vi "AlliGator Update Settings Python Options & Valid Flag.vi"(8 "error in (no error)":errorcluster, 11 "Ctl Refnums":refnum<vi>[](array[refnum])) -> (0 "error out":errorcluster)   [LabVIEW 2021, in "AlliGator Settings.lvlib"]
doc: "Updates Python Plugins options and Valid Session flag in the Settings window."
uses:
  AlliGator Settings.lvlib
  AlliGator Python Settings.ctl
  AlliGator Variables List.ctl
  Variant/Variant to Data/Variant to Boolean.vi
  AlliGator Globals, Variables & Constants.lvlib
  Variant/Variant to Data/Variant to Data.lvlib
panel:
  out "Valid Python Session":bool
  in  "Python Settings":T1
  # "see the AlliGator License on the block diagram (Ctrl+E or Window:Show Block Diagram)"
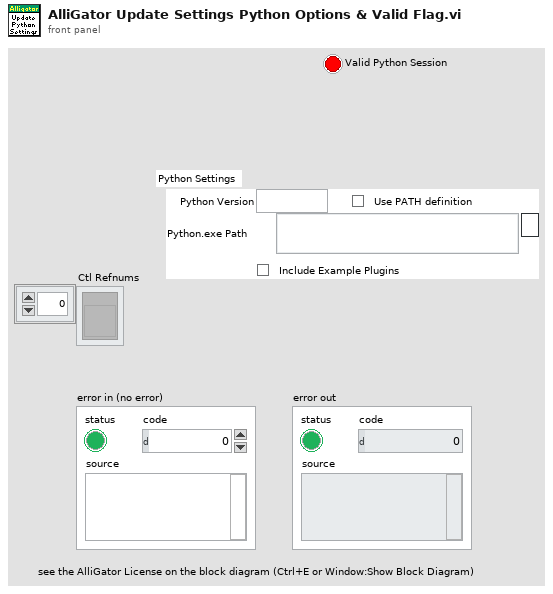
[diagram p1: front panel]
types:
  T1 = typedef "AlliGator Settings.lvlib/AlliGator Python Settings.ctl" = cluster{"Python Version":string, "Use PATH definition":bool, "Python.exe Path":path, "Include Example Plugins":bool}
  T2 = typedef "AlliGator Globals, Variables & Constants.lvlib/AlliGator Variables List.ctl" = enum16{"---- GUI ----", "Initialization Status", "State Indicators Refnum", "Original AlliGator Menu Items", "Current Action Loop State", "Script in progress", "Playback", "Loop Playback", "Search ROI Used", "Search ROI", "Decay Graph Max Legend Size", "Intensity Graph Max Legend Size", "Decay Statistics Graph Max Legend Size", "Phasor Graph Max Legend Size", "Phasor Ratio Graph Max Legend Size", "Lifetime Graph Max Legend Size", "---- Files ----", "Export Dataset Frames as Individual Files", "Show Batch Export Help Balloons", "Frames in Dataset", "ptu File Frame Start Indices", "Current Frame in Dataset", "Current Frame Timestamp", "------ Python Plugins ------", "Python Plugins Information", "Python Session", "Valid Python Session?", "---- Source Image ----", "Dataset Loaded", "Dataset Metadata", "Dataset Channel", "Dataset Data Description", "Background Dataset Metadata", "Background Dataset Channel", "Background Dataset Data Description", "Background File Subtraction", "Background File Path", "Background File Pile-up Correction", "Background File Pixel Well Capacity", "Background File Scaling Factor", "Source Image ROIs", "Current Source Image ROI", "Source Image ROI Event Refnum", "X_Source Image Display Range", "X_Source Image Palette Information", "Source Image Palette List", "Source Image Scale", "Current Dataset Load Settings", "Source Image:ROI Overlay Color", "---- Image Profile Window ----", "Image Profile:Overlay ROI in Source Image", "Image Profile Window Event Refnum", "Image Profile:IntensityType", "Image Profile:Intensity Average Type", "Image Profile:Intensity-weighted SDV", "Image Profile:Box Profile Type", "Image Profile Window Open", "Image Profile:Plotted Fit Parameter", "X_Type of Displayed Image", "X_Time Gate Slider", "Dataset Path", "Source Image Overlay to Erase", "Is Displayed Image Accumulated", "White Light Image Modified", "Mask Image Modified", "Macrotime Gate Separation", "------ Phasor Graph -------", "Phasor Graph:Show Line", "---- Phasor Plot ---", "Phasor Plot Parameters Changed", "FLI Dataset Modified since last Phasor Plot Calculation", "Phasor Harmonics Data", "Selected Phasor Harmonics", "Phasor Harmonic Manager Event Refnum", "Phasor Plot ROIs", "Current Phasor Plot ROI", "Phasor Plot ROI Event Refnum", "Phasor Plot Image Reference Points", "Phasor Plot Computed", "Phasor Plot Palette Information", "Phasor Plot Palette List", "Phasor Ratio Palette Information", "Phasor Ratio Palette List", "Phasor Image Scale", "Phasor Plot Image Overlay to Erase", "Phasor Plot Image Elements to Update", "Current Phasor Plot Calculation Parameters", "Current Phasor Calibration Options", "Reset Cumulated Phasor Plot", "Phasor Ratio Reference 1", "Phasor Ratio Lifetime Reference 1", "Phasor Ratio Reference 1 Frequency", "Phasor Ratio Reference 2", "Phasor Ratio Lifetime Reference 2", "Phasor Ratio Reference 2 Frequency", "---- Decay Analysis ----", "Number of Selected Decays to Fit", "LS Fit Results", "LAR Fit Results", "BS Fit Results", "Last Decay Max - Min", "Best Fit Parameters", "Best Fit Parameter Names", "Actual Size X", "Actual Size Y", "Binning X", "Binning Y", "Actual # Gates", "Dataset Number", "Gates to...", "Gates Skipped", "Gates to keep", "Gate Step", "Gate Separation", "Reversed Gates", "Pile-up Correction", "Pixel Well Capacity", "Background Subtracted", "Background Subtraction Method", "Background Definition Range", "Background File (deprecated)", "Number of Dataset Accumulated", "Array of Accumulated Dataset Paths", "Do Averaged Datasets", "Destination File Path", "Process Plot Target", "Use 1/D as Phasor Frequency", "---- Decay Fit Parameter Map -----", "Decay Fit Parameter Map Palette Information", "Decay Fit Parameter Map Palette List", "Local Decay Graph Window Event Refnum", "------- Local Decay Window ---------", "Use normalized IRF for convolution", "----- Miscellaneous ----", "Skippable Dialog Windows Status"}
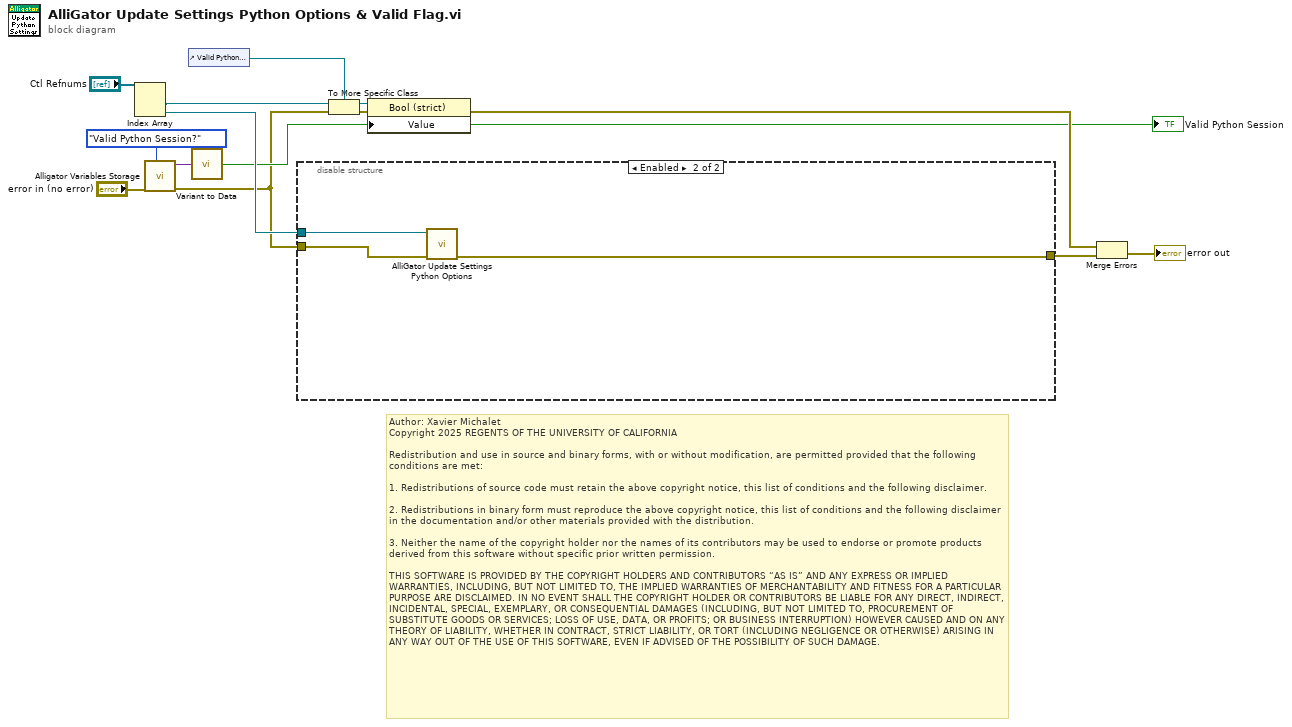
[diagram p0: block diagram]
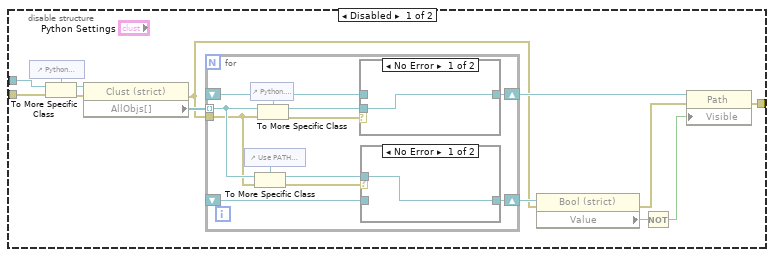
[diagram p2: hidden frame]
diagram:
  # "Author: Xavier Michalet\nCopyright 2025 REGENTS OF THE UNIVERSITY OF CALIFORNIA\n\nRedistribution and use in source and binary forms, with or without modification, are permitted provided that the following conditions are met:\n\n1. Redistributions of source code must retain the above copyright notice, this list of conditions and the following disclaimer.\n\n2. Redistributions in binary form must reproduce the above copyright notice, this list of conditions and the following disclaimer in the documentation and/or other materials provided with the distribution.\n\n3. Neither the name of the copyright holder nor the names of its contributors may be used to endorse or promote products derived from this software without specific prior written permission.\n\nTHIS SOFTWARE IS PROVIDED BY THE COPYRIGHT HOLDERS AND CONTRIBUTORS “AS IS” AND ANY EXPRESS OR IMPLIED WARRANTIES, INCLUDING, BUT NOT LIMITED TO, THE IMPLIED WARRANTIES OF MERCHANTABILITY AND FITNESS FOR A PARTICULAR PURPOSE ARE DISCLAIMED. IN NO EVENT SHALL THE COPYRIGHT HOLDER OR CONTRIBUTORS BE LIABLE FOR ANY DIRECT, INDIRECT, INCIDENTAL, SPECIAL, EXEMPLARY, OR CONSEQUENTIAL DAMAGES (INCLUDING, BUT NOT LIMITED TO, PROCUREMENT OF SUBSTITUTE GOODS OR SERVICES; LOSS OF USE, DATA, OR PROFITS; OR BUSINESS INTERRUPTION) HOWEVER CAUSED AND ON ANY THEORY OF LIABILITY, WHETHER IN CONTRACT, STRICT LIABILITY, OR TORT (INCLUDING NEGLIGENCE OR OTHERWISE) ARISING IN ANY WAY OUT OF THE USE OF THIS SOFTWARE, EVEN IF ADVISED OF THE POSSIBILITY OF SUCH DAMAGE."
  n1 = Index Array(array="Ctl Refnums") -> (element #1=w7:refnum<vi>, element #2=w14:refnum<vi>)  [unwired: 2 in]
  n2 = call "Alligator Variables Storage.vi"("AlliGator Variable"=AlliGator_Variables_List."Valid Python Session?" ("Alligator Variable"), "Error In"="error in (no error)") -> ("Error Out"=w1:errorcluster, "Data out"=w6:variant)  [unwired: 7 in, 1 out]
  n3 = control-ref of="Valid Python Session"() -> (w4:refnum<vi>)
  n4 = call-poly "Variant to Data.vi"("Variant"=w6) -> ("Value"=w2:bool)  [unwired: 8 in]
  "Valid Python Session" <- w2
  n5 = disable-structure shown="Enabled" {
    disable-tunnel: w14 -> [w26 w46]
    disable-tunnel: [w18 w44] -> w3
    disable-tunnel: w1 -> [w16 w45]
    frame Disabled {
      n6 = control-ref of="Python Settings"() -> (w25:refnum<vi>)
      n7 = To More Specific Class(target class=w25, reference=w26, error in=w16) -> (specific class reference=w27:refnum<vi>, error out=w24:errorcluster)
      n8 = property class="Clust (strict)"(reference=w27, error in=w24) -> (error out=w15:errorcluster, "AllObjs[]"=w23:refnum<vi>[])  [unwired: 1 out]
      n9 = for {
        tunnel: w23 -> [w34] mode=indexing
        shift-right: [w37] -> w22
        shift-left: _ -> [w30]
        shift-right: [w32] -> w21
        shift-left: _ -> [w29]
        tunnel: w15 -> [w28]
        n10 = control-ref of="Use PATH definition"() -> (w35:refnum<vi>)
        n11 = control-ref of="Python.exe Path"() -> (w39:refnum<vi>)
        n12 = To More Specific Class(target class=w35, reference=w34, error in=w28) -> (specific class reference=w31:refnum<vi>, error out=w33:errorcluster)
        n13 = To More Specific Class(target class=w39, reference=w34, error in=w28) -> (specific class reference=w36:refnum<vi>, error out=w38:errorcluster)
        n14 = case shown="No Error" w38 {
          tunnel: [w42 w43] -> w37
          tunnel: w36 -> [w42 _]
          tunnel: w30 -> [_ w43]
          frame No Error {
          }
          frame Error {
          }
        }
        n15 = case shown="No Error" w33 {
          tunnel: [w40 w41] -> w32
          tunnel: w31 -> [w40 _]
          tunnel: w29 -> [_ w41]
          frame No Error {
          }
          frame Error {
          }
        }
      }
      n16 = property class="Bool (strict)"(reference=w21, error in=w15) -> (error out=w19:errorcluster, "Value"=w20:bool)  [unwired: 1 out]
      n17 = Not(x=w20) -> (.not. x?=w17:bool)
      n18 = property class="Path"(reference=w22, error in=w19, "Visible"=w17) -> (error out=w18:errorcluster)  [unwired: 1 out]
    }
    frame Enabled {
      n19 = call "AlliGator Update Settings Python Options.vi"("error in (no error)"=w45, "Python Settings Refnum"=w46) -> ("error out"=w44:errorcluster)  [unwired: 9 in]
    }
  }
  n20 = To More Specific Class(target class=w4, reference=w7, error in=w1) -> (specific class reference=w9:refnum<vi>, error out=w10:errorcluster)
  n21 = property class="Bool (strict)"(reference=w9, error in=w10, "Value"=w2) -> (error out=w11:errorcluster)  [unwired: 1 out]
  n22 = Merge Errors(w11, w3) -> (→"error out":errorcluster)
